vi "Dispose.vi"(0 "reference in":refnum<class "ConveyorBelt.lvclass">, 5 "error in (no error)":errorcluster) -> (14 "reference out":refnum<class "ConveyorBelt.lvclass">, 19 "error out":errorcluster)   [LabVIEW 2014, in "ConveyorBelt.lvclass"]
uses:
  ConveyorBelt.lvclass
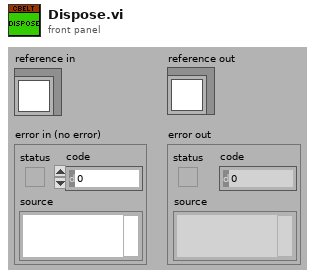
[diagram p1: front panel]
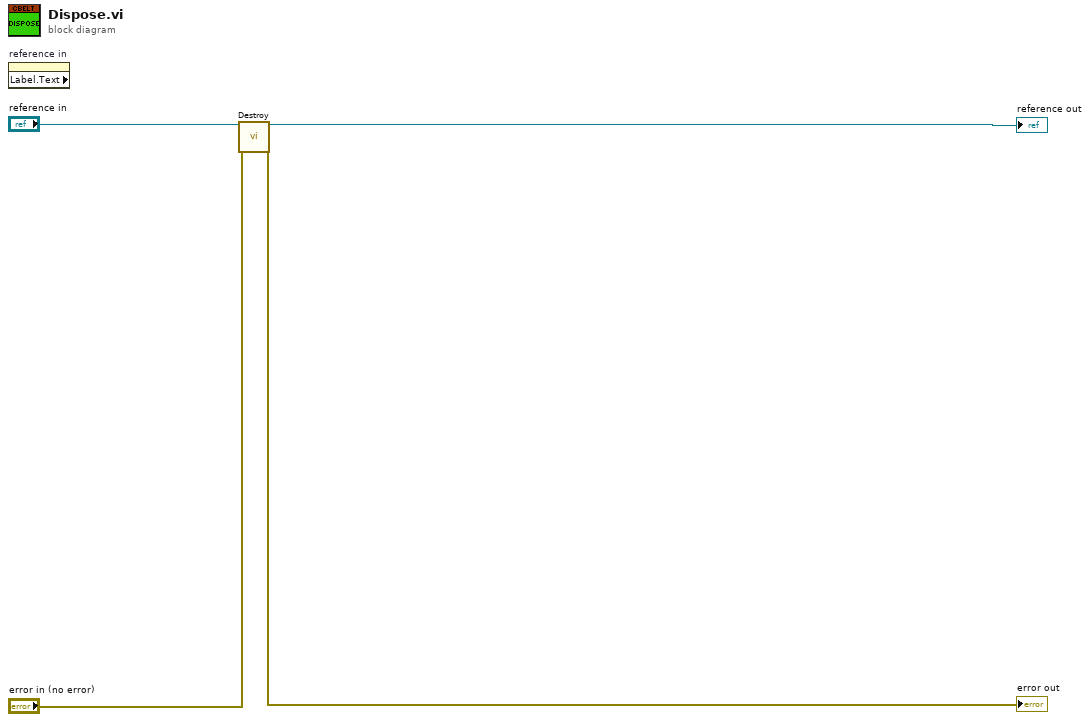
[diagram p0: block diagram]
diagram:
  n1 = property on="reference in" class="LVClassControl (strict)" props=["Label", "Text"]() -> ()  [unwired: 2 in, 3 out]
  n2 = call-dynamic "Destroy.vi"("reference in"="reference in", "error in (no error)"="error in (no error)") -> ("reference out"=→"reference out":refnum<class "ConveyorBelt.lvclass">, "error out"=→"error out":errorcluster)  [unwired: 16 in]
